vi "Get Section Relays.vi"(8 "error in (no error)":errorcluster, 11 "MUX Section Ref in":T1 format="%.0x") -> (0 "error out":errorcluster, 2 "Section Relays Array":T2[](array[typedef]), 3 "MUX Section Ref out":T1=18446744073709551615 format="%.0x")   [LabVIEW 2013, in "MUX Custom Device.lvlib"]
uses:
  MUX Custom Device.lvlib
  <vilib>/NI Veristand/Custom Device API/Custom Device Item Ref.ctl
  Relay Data.ctl
  Switch.ctl
  MUX Global.vi
  <vilib>/NI Veristand/Custom Device API/Get Item Property (String).vi
  <vilib>/NI Veristand/Custom Device API/Custom Device API.lvlib
  <vilib>/NI Veristand/Custom Device Tools/Custom Device Utility Library/Custom Device Utility Library.lvlib
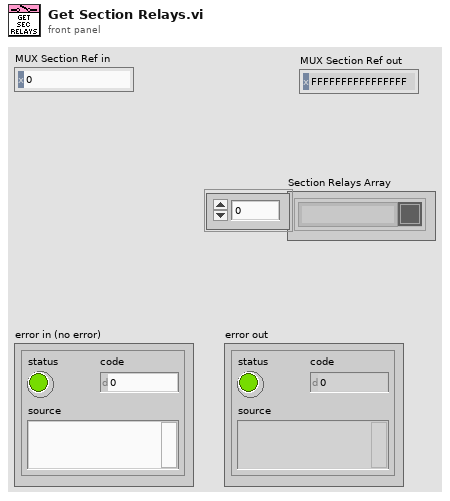
[diagram p1: front panel]
types:
  T1 = typedef "Custom Device API.lvlib/Custom Device Item Ref.ctl" = u64
  T2 = typedef "MUX Custom Device.lvlib/Relay Data.ctl" = cluster{"Relay Name":string, "State":T3}
  T3 = typedef "MUX Custom Device.lvlib/Switch.ctl" = bool
  T4 = typedef "Custom Device API.lvlib/Custom Device Channel.ctl" = cluster{"Type":T5, "Units":string, "Default Value":dbl, "Faultable":bool, "Scalable":bool}
  T5 = typedef "Custom Device API.lvlib/Custom Device Channel Type.ctl" = enum16{"Input", "Output"}
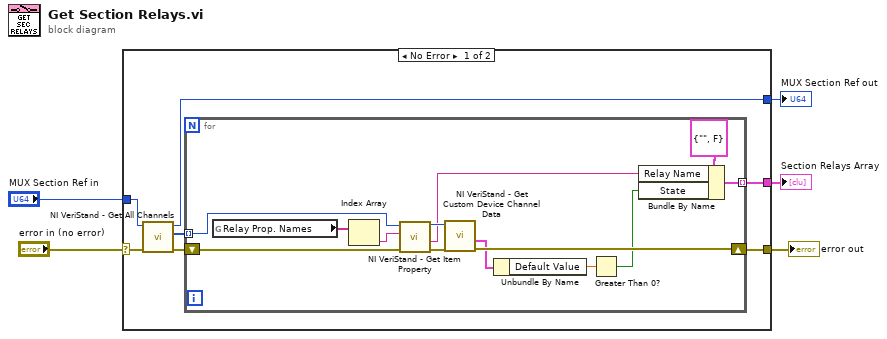
[diagram p0: block diagram]
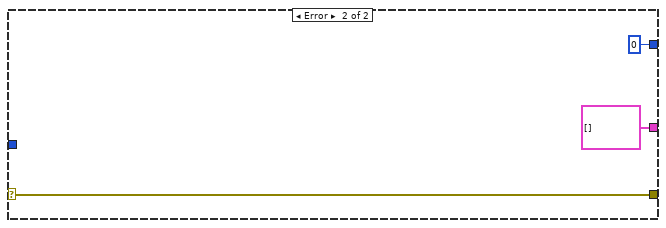
[diagram p2: hidden frame]
diagram:
  n1 = case shown="No Error" "error in (no error)" {
    selector: "error in (no error)" -> [w12 w28]
    tunnel: "MUX Section Ref in" -> [w11 _]
    tunnel: [w9 w28] -> w5
    tunnel: [w8 T2[] []] -> w2
    tunnel: [w6 T1 0 ("Section Ref out")] -> w1
    frame No Error {
      n2 = call <vilib>:"NI VeriStand - Get All Channels.vi"("error in"=w12, "Section Ref in"=w11) -> ("error out"=w10:errorcluster, "Channel Refs"=w7:T1[], "Section Ref out"=w6:T1)  [unwired: 6 in, 1 out]
      n3 = for {
        tunnel: w7 -> [w25] mode=indexing
        shift-right: [w20] -> w9
        shift-left: w10 -> [w22]
        tunnel: [w13] -> w8 mode=indexing
        n4 = global read "MUX Global.vi" "Relay Prop. Names"() -> (w24:string[])
        n5 = Index Array(array=w24) -> (element=w23:string)  [unwired: 1 in]
        n6 = call-poly <vilib>:"NI VeriStand - Get Item Property.vi"("error in (no error)"=w22, "Property Name"=w23, "Item Ref in"=w25) -> ("error out"=w21:errorcluster, "Value"=w15:string, "Item Ref out"=w19:T1)  [unwired: 5 in, 1 out]
        n7 = call <vilib>:"NI VeriStand - Get Custom Device Channel Data.vi"("error in (no error)"=w21, "Channel Ref in"=w19) -> ("error out"=w20:errorcluster, "Channel"=w18:T4)  [unwired: 4 in, 4 out]
        n8 = Unbundle By Name(w18) -> ("Default Value"=w17:dbl)
        n9 = Greater Than 0?(x=w17) -> (x > 0?=w14:bool)
        n10 = Bundle By Name(cluster=T2 {"Relay Name"="", "State"=FALSE} ("Relay Data"), "Relay Name"=w15, "State"=w14) -> (w13:T2)
      }
    }
    frame Error {
    }
  }
  "error out" <- w5
  "Section Relays Array" <- w2
  "MUX Section Ref out" <- w1
